vi "2 Don't Flip Setpoints - Olli.vi"() -> (0 "Setpoint Cluster":T3)   [LabVIEW 2011]
doc: "This VI simply outputs constant sail and rudder setpoints with priority set by the input. These setpoints will be used if no other higher priority think function outputs true priority.\nThis VI takes over control as soon as the boat is over an angle of 45/ -45 degrees.\nDepending on the wind direction, the sail will be taken out of the wind, causing the boat to flip back.\nDuring that time, the Rudder is locked to 0 deg, to avoid turning further into the wind."
uses:
  2 Typedefs/setpoints to arbiter.ctl
  2 Typedefs/pitch and roll.ctl
  2 Typedefs/absolute wind direction.ctl
  2 Typedefs/apparent wind direction.ctl
  2 Globals/2 Global.vi
panel:
  out "Tipping?":bool
  in  "Roll":dbl
  in  "Absolute Wind\nDirection (º)":T1
  in  "Manual input\n(instead of global)":bool
  out "Robot Pitch/Roll\nfrom Global":T2 {"Roll" format="%05.1f"; "Pitch" format="%05.1f"}
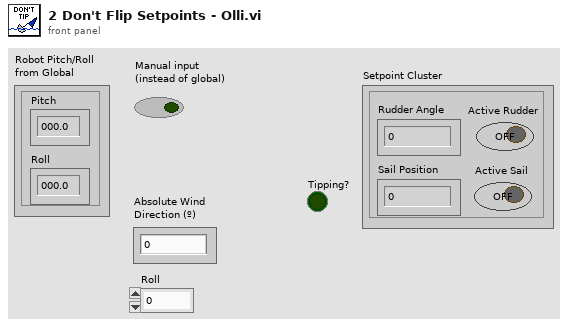
[diagram p1: front panel]
types:
  T1 = typedef "absolute wind direction.ctl" = dbl
  T2 = typedef "pitch and roll.ctl" = cluster{"Pitch":dbl, "Roll":dbl}
  T3 = typedef "setpoints to arbiter.ctl" = cluster{"Rudder Angle":dbl, "Sail Position":dbl, "Active Rudder":bool, "Active Sail":bool}
  T4 = typedef "apparent wind direction.ctl" = dbl
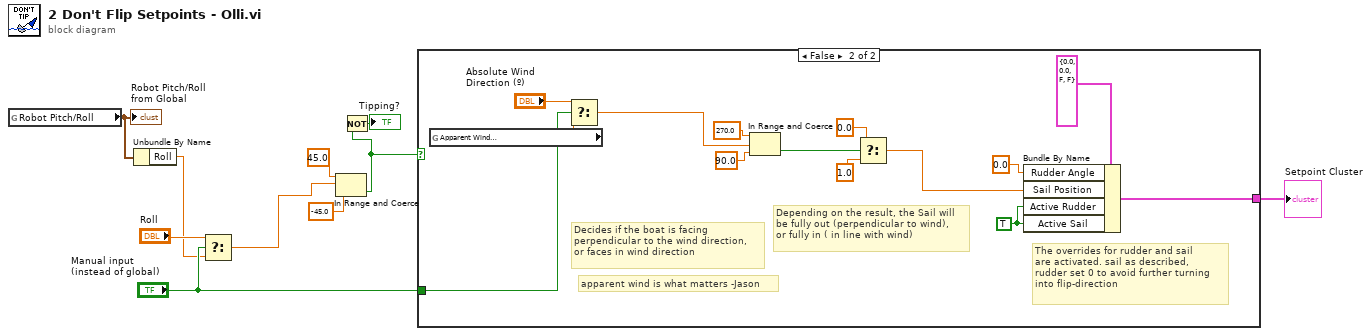
[diagram p0: block diagram]
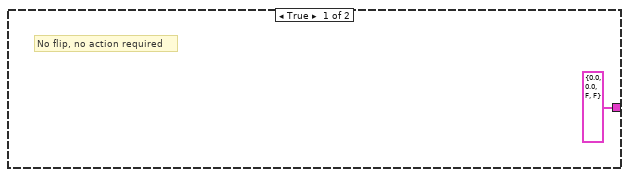
[diagram p2: hidden frame]
diagram:
  n1 = global read "2 Global.vi" "Robot Pitch/Roll"() -> (w10:T2)
  "Robot Pitch/Roll\nfrom Global" <- w10
  n2 = Unbundle By Name(w10) -> ("Roll"=w4:dbl)
  n3 = Select(t="Roll", s="Manual input\n(instead of global)", f=w4) -> (s? t:f=w3:dbl)
  n4 = In Range and Coerce(upper limit=45.0, x=w3, lower limit=-45.0) -> (In Range?=w1:bool)  [unwired: 1 out]
  n5 = Not(x=w1) -> (.not. x?=→"Tipping?":bool)
  n6 = case shown="False" w1 {
    tunnel: [T3 {"Rudder Angle"=0.0, "Sail Position"=0.0, "Active Rudder"=FALSE, "Active Sail"=FALSE} ("Setpoint Cluster") w20] -> w7
    tunnel: "Manual input\n(instead of global)" -> [_ w16]
    frame True {
      # "No flip, no action required"
    }
    frame False {
      w19 = TRUE ("Use Defaults")
      # "apparent wind is what matters -Jason"
      # "The overrides for rudder and sail \nare activated. sail as described,\nrudder set 0 to avoid further turning \ninto flip-direction"
      # "Depending on the result, the Sail will\nbe fully out (perpendicular to wind),\nor fully in ( in line with wind)"
      # "Decides if the boat is facing \nperpendicular to the wind direction,\nor faces in wind direction"
      n7 = global read "2 Global.vi" "Apparent Wind\nDirection (º)"() -> (w17:T4)
      n8 = Select(t="Absolute Wind\nDirection (º)", s=w16, f=w17) -> (s? t:f=w15:T4)
      n9 = In Range and Coerce(upper limit=T4 270.0, x=w15, lower limit=T4 90.0) -> (In Range?=w12:bool)  [unwired: 1 out]
      n10 = Select(t=0.0, s=w12, f=1.0) -> (s? t:f=w21:dbl)
      n11 = Bundle By Name(cluster=T3 {"Rudder Angle"=0.0, "Sail Position"=0.0, "Active Rudder"=FALSE, "Active Sail"=FALSE} ("Setpoint Cluster"), "Rudder Angle"=0.0, "Sail Position"=w21, "Active Rudder"=w19, "Active Sail"=w19) -> (w20:T3)
    }
  }
  "Setpoint Cluster" <- w7
